vi "rad_FilterTargets.vi"(8 "error in (no error)":errorcluster, 10 "Target Types":string[](array[string]), 11 "Targets Information":T1[](array[typedef]) {"Primary NIC"."IP Address Request Mode" items=["Static"=1, "DHCP/Link-Local"=2, "Link-Local Only"=4, "DHCP Only"=8]}) -> (0 "error out":errorcluster, 1 "Filtered Targets":i32[](array[numeric]), 3 "Targets Information":T1[](array[typedef]) {"Primary NIC"."IP Address Request Mode" items=["Static"=1, "DHCP/Link-Local"=2, "Link-Local Only"=4, "DHCP Only"=8]})   [LabVIEW 2020]
uses:
  Target Information.ctl
  subVIs/Targets/TypeDefs/rad_Target Network Settings.ctl
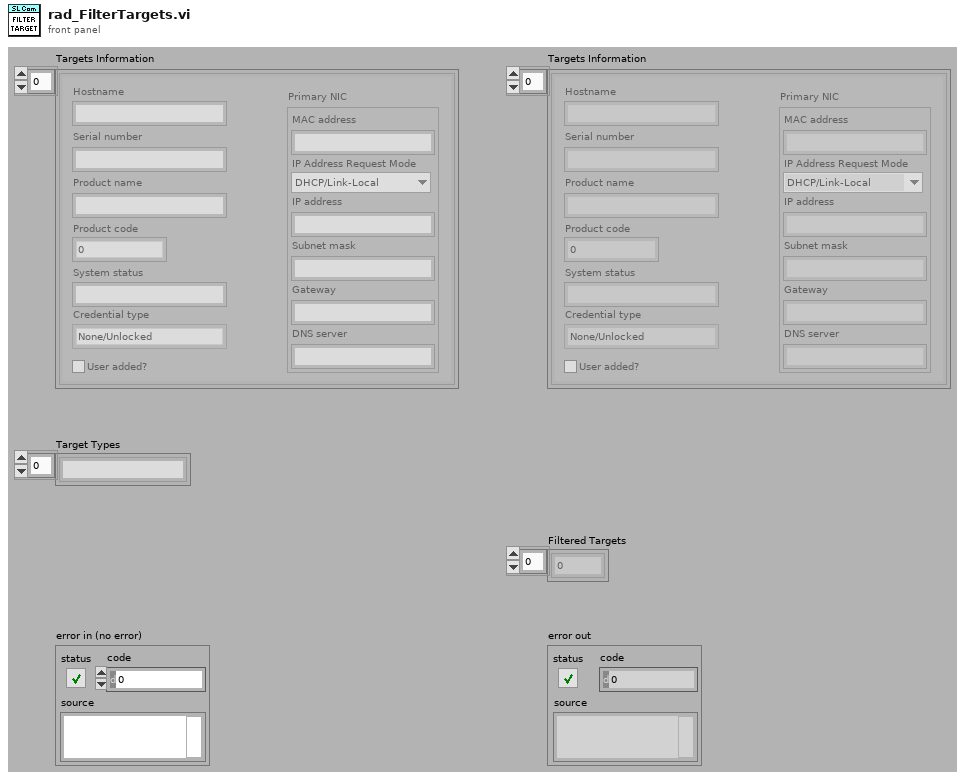
[diagram p1: front panel]
types:
  T1 = typedef "Target Information.ctl" = cluster{"Hostname":string, "Serial number":string, "Product name":string, "Product code":i32, "System status":string, "Credential type":enum16{"None/Unlocked", "FTP Password", "NIAuth Credentials"}, "User added?":bool, "Primary NIC":T2}
  T2 = typedef "rad_Target Network Settings.ctl" = cluster{"MAC address":string, "IP Address Request Mode":i32, "IP address":string, "Subnet mask":string, "Gateway":string, "DNS server":string}
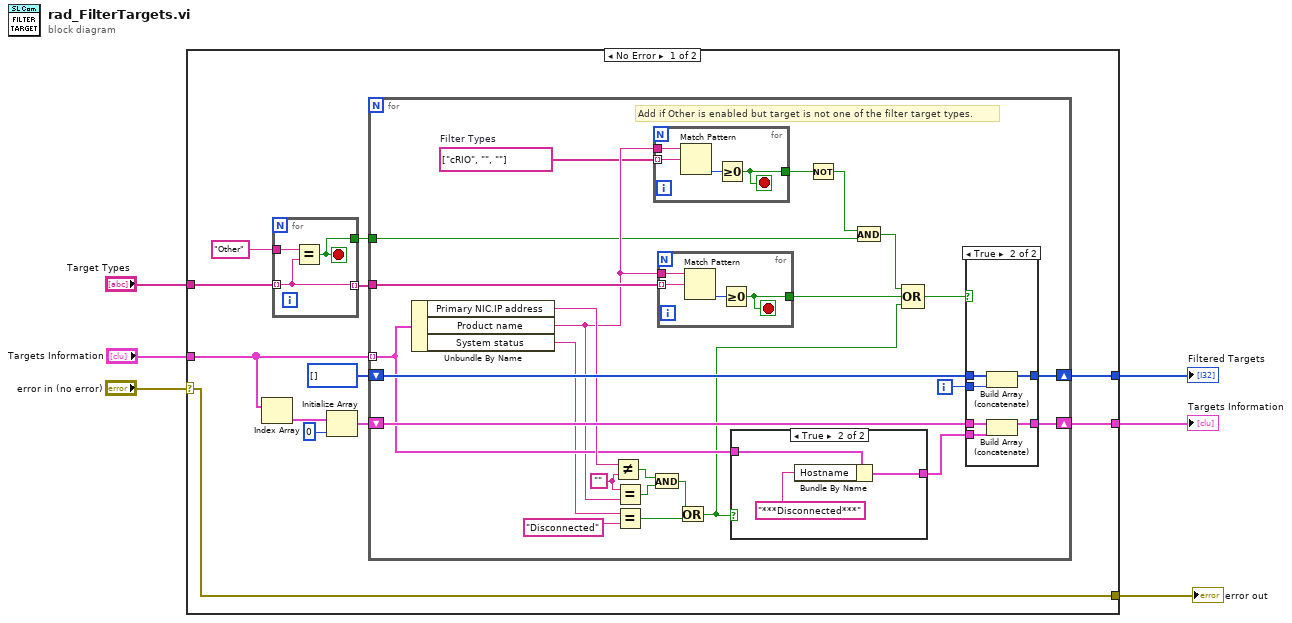
[diagram p0: block diagram]
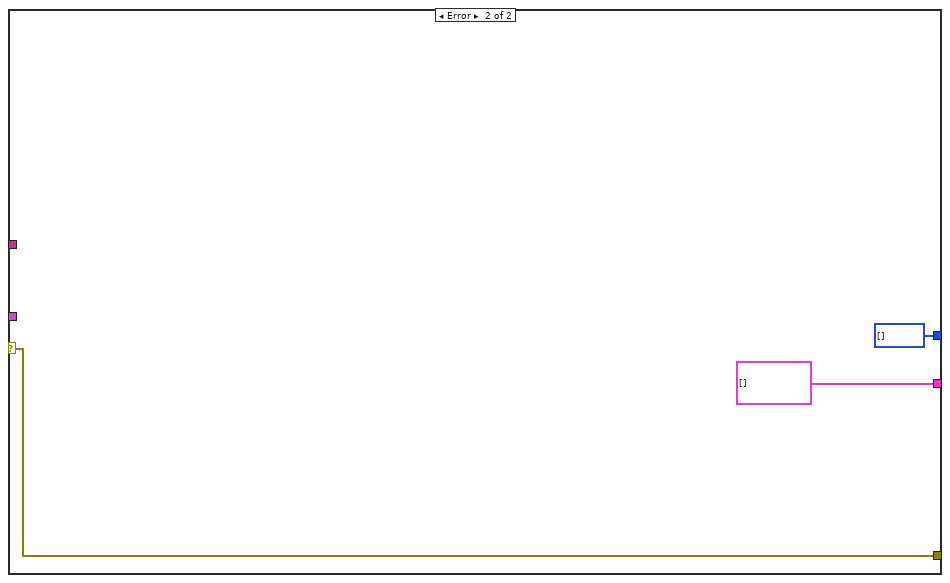
[diagram p4: hidden frame]
diagram:
  n1 = case shown="No Error" "error in (no error)" {
    selector: "error in (no error)" -> [w7 w69]
    tunnel: "Targets Information" -> [w15 _]
    tunnel: [w14 T1[] []] -> w5
    tunnel: [w12 i32[] []] -> w4
    tunnel: "Target Types" -> [w11 _]
    tunnel: [w7 w69] -> w1
    frame No Error {
      n2 = Index Array(array=w15) -> (element=w17:T1)  [unwired: 1 in]
      n3 = for {
        tunnel: w11 -> [w20] mode=indexing
        tunnel: [w20] -> w10 mode=indexing
        tunnel: "Other" ("y") -> [w19]
        tunnel: [w21] -> w8
        stop <- w21 stop-if-true
        n4 = Equal?(x=w19, y=w20) -> (x = y?=w21:bool)
      }
      n5 = Initialize Array(w17, 0 ("dimension size")) -> (w16:T1[])
      n6 = for {
        shift-right: [w45] -> w14
        shift-left: w16 -> [w46]
        tunnel: w15 -> [w35] mode=indexing
        tunnel: w10 -> [w44]
        shift-right: [w42] -> w12
        shift-left: i32[] [] -> [w41]
        tunnel: w8 -> [w23]
        i -> [w43]
        w26 = string[] ["cRIO", "", ""]  # Filter Types
        w39 = ""
        # "Add if Other is enabled but target is not one of the filter target types."
        n7 = Unbundle By Name(w35) -> ("Primary NIC.IP address"=w40:string, "Product name"=w27:string, "System status"=w33:string)
        n8 = Not Equal?(x=w40, y=w39) -> (x != y?=w38:bool)
        n9 = Equal?(x=w39, y=w27) -> (x = y?=w37:bool)
        n10 = Equal?(x=w33, y="Disconnected") -> (x = y?=w30:bool)
        n11 = And(x=w38, y=w37) -> (x .and. y?=w31:bool)
        n12 = for {
          tunnel: w27 -> [w50]
          tunnel: w26 -> [w49] mode=indexing
          tunnel: [w47] -> w25
          stop <- w47 stop-if-true
          n13 = Match Pattern(string=w50, regular expression=w49) -> (offset past match=w48:i32)  [unwired: 4 out]
          n14 = Greater Or Equal To 0?(x=w48) -> (x >= 0?=w47:bool)
        }
        n15 = for {
          tunnel: w27 -> [w58]
          tunnel: w44 -> [w57] mode=indexing
          tunnel: [w55] -> w28
          stop <- w55 stop-if-true
          n16 = Match Pattern(string=w58, regular expression=w57) -> (offset past match=w56:i32)  [unwired: 4 out]
          n17 = Greater Or Equal To 0?(x=w56) -> (x >= 0?=w55:bool)
        }
        n18 = Or(x=w31, y=w30) -> (x .or. y?=w29:bool)
        n19 = case shown="True" w29 {
          tunnel: w35 -> [w51 w54]
          tunnel: [w51 w52] -> w34
          frame False {
          }
          frame True {
            n20 = Bundle By Name(cluster=w54, "Hostname"="***Disconnected***" ("IP settings.DNS name")) -> (w52:T1)
          }
        }
        n21 = Not(x=w25) -> (.not. x?=w24:bool)
        n22 = And(x=w24, y=w23) -> (x .and. y?=w22:bool)
        n23 = Compound Arithmetic op=OR(w22, w28, w29) -> (w36:bool)
        n24 = case shown="True" w36 {
          tunnel: w46 -> [w60 w66]
          tunnel: [w60 w64] -> w45
          tunnel: w34 -> [_ w65]
          tunnel: w43 -> [_ w63]
          tunnel: [w59 w62] -> w42
          tunnel: w41 -> [w59 w61]
          frame False {
          }
          frame True {
            n25 = Build Array (concatenate)(w61, w63) -> (w62:i32[])
            n26 = Build Array (concatenate)(w66, w65) -> (w64:T1[])
          }
        }
      }
    }
    frame Error {
    }
  }
  "Targets Information" <- w5
  "Filtered Targets" <- w4
  "error out" <- w1
